vi "GetProjectPath.vi"() -> (1 "ProjectRootPath":path, 3 "LvProjectPath":path)   [LabVIEW 2020]
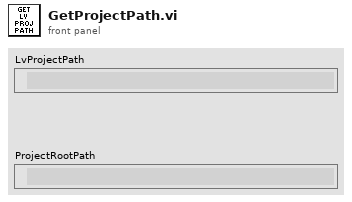
[diagram p1: front panel]
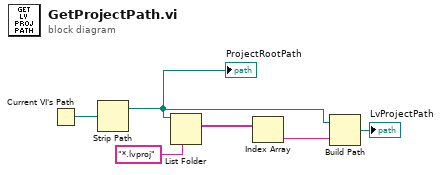
[diagram p0: block diagram]
diagram:
  n1 = Current VI's Path() -> (path=w6:path)
  n2 = Strip Path(path=w6) -> (stripped path=w3:path)  [unwired: 1 out]
  "ProjectRootPath" <- w3
  n3 = List Folder(path=w3, pattern="*.lvproj") -> (filenames=w4:string[])  [unwired: 2 in, 3 out]
  n4 = Index Array(array=w4) -> (element=w2:string)  [unwired: 1 in]
  n5 = Build Path(base path=w3, name or relative path=w2) -> (appended path=→"LvProjectPath":path)
